vi "Initialize.vi"(8 "error in (no error)":errorcluster, 11 "GPIB in":refnum<class "GPIB.lvclass">=refnum) -> (0 "error out":errorcluster, 3 "GPIB out":refnum<class "GPIB.lvclass">)   [LabVIEW 2019, in "GPIB.lvclass"]
uses:
  GPIB.lvclass
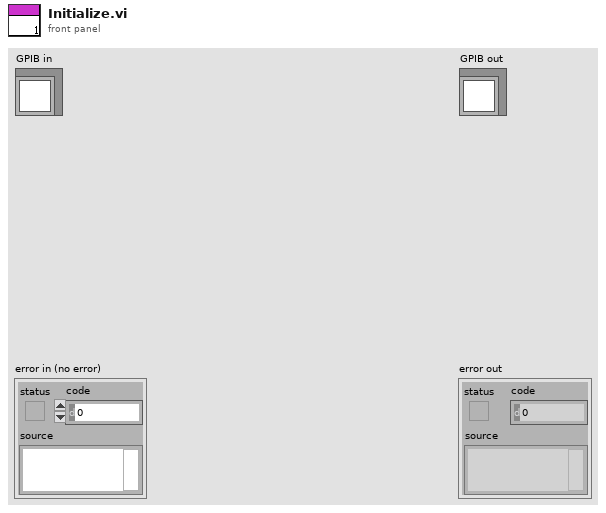
[diagram p1: front panel]
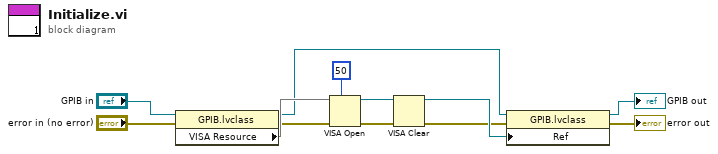
[diagram p0: block diagram]
diagram:
  n1 = property class="GPIB.lvclass"(reference="GPIB in", error in="error in (no error)") -> (reference out=w7:refnum<class "GPIB.lvclass">, error out=w8:errorcluster, "VISA Resource"=w10)
  n2 = VISA Open(timeout (0)=u32 50 ("VISA Open timeout (0)"), error in (no error)=w8, VISA resource name=w10) -> (VISA resource name=w4:refnum<visa-resource-name>, error out=w2:errorcluster)  [unwired: 2 in]
  n3 = VISA Clear(VISA resource name=w4, error in (no error)=w2) -> (VISA resource name out=w3:refnum<visa-resource-name>, error out=w1:errorcluster)
  n4 = property class="GPIB.lvclass"(reference=w7, error in=w1, "Ref"=w3) -> (reference out=→"GPIB out":refnum<class "GPIB.lvclass">, error out=→"error out":errorcluster)
